vi "OE2052_USB_Query Data.vi"(0 "VISA resource name":refnum<visa-resource-name>, 11 "Error in (no error)":errorcluster caption="error out（no error）") -> (3 "Buffer Count":u8, 4 "VISA resource  out":refnum<visa-resource-name>, 6 "Parameter Values":T1, 8 "Total Data Array":dbl[][](array[numeric]), 10 "Output String":string, 14 "A&B_PLL&Overload":T2, 15 "Error out":errorcluster caption="error out")   [LabVIEW 2011]
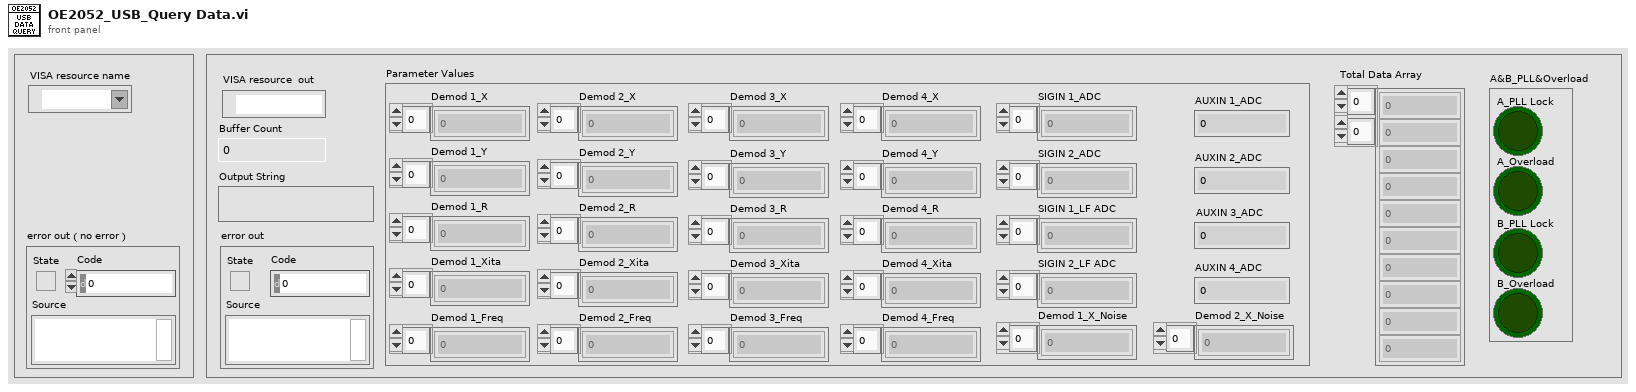
[diagram p1: front panel]
types:
  T1 = cluster{"Demod 1_X":dbl[], "Demod 1_Y":dbl[], "Demod 1_R":dbl[], "Demod 1_Xita":dbl[], "Demod 1_Freq":dbl[], "Demod 2_X":dbl[], "Demod 2_Y":dbl[], "Demod 2_R":dbl[], "Demod 2_Xita":dbl[], "Demod 2_Freq":dbl[], "Demod 3_X":dbl[], "Demod 3_Y":dbl[], "Demod 3_R":dbl[], "Demod 3_Xita":dbl[], "Demod 3_Freq":dbl[], "Demod 4_X":dbl[], "Demod 4_Y":dbl[], "Demod 4_R":dbl[], "Demod 4_Xita":dbl[], "Demod 4_Freq":dbl[], "SIGIN 1_ADC":dbl[], "SIGIN 2_ADC":dbl[], "SIGIN 1_LF ADC":dbl[], "SIGIN 2_LF ADC":dbl[], "AUXIN 1_ADC":dbl, "AUXIN 2_ADC":dbl, "AUXIN 3_ADC":dbl, "AUXIN 4_ADC":dbl, "Demod 1_X_Noise":dbl[], "Demod 2_X_Noise":dbl[]}
  T2 = cluster{"A_PLL Lock":bool, "A_Overload":bool, "B_PLL Lock":bool, "B_Overload":bool}
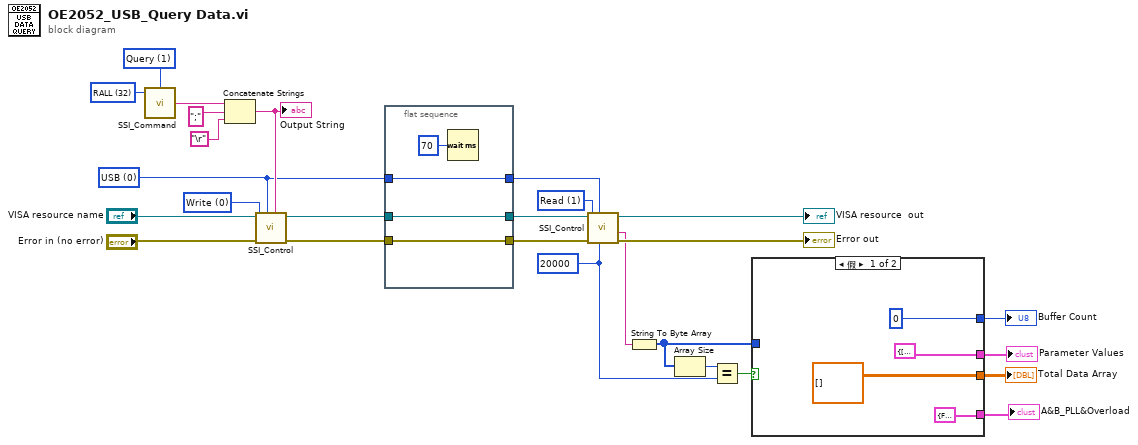
[diagram p0: block diagram]
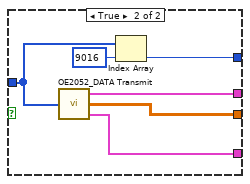
[diagram p2: hidden frame]
diagram:
  w3 = u16 0 items=["USB"=0, "RS232"=1, "Ethernet"=3] ("Remote Mode")
  w14 = u32 20000 ("Number of bytes")
  w17 = u16 1 items=["Write", "Read"] ("Control")
  w19 = u16 0 items=["Write", "Read"] ("Control")
  w24 = u16 32 items=["ISRC", "IGND", "ICPL", "ILIN", "PHAS", "FMOD", "RSLP", "FREQ", "SWPT", "SLLM", "SULM", "SSLL", "SSLG", "STLM", "SWRM", "IRNG", "SENS", "RMOD", "OFLT", "OFSL", "SYNC", "DMOD", "HARM", "DARB", "SWVT", "SLVL", "SVLL", "SVUL", "SVSL", "SVSG", "SVTM", "SVRM", "RALL", "SNAP", "OUTP", "OAUX", "COUT", "CAUX", "COFP", "CEXP", "FPOP", "OEXP", "*IDN", "*RST", "OVLD", "INOV", "GNOV", "*PLL", "SSET", "RSET", "AGAN", "APHS", "ARSV", "ASCL", "EQCD", "EQCS", "SPED", "SRAT", "SLEN", "SSLE", "STRG", "SPRM", "STRD", "PAUS", "RSET", "SPTS", "TRCA", "TEMP", "RSTU", "INHZ", "DEQU", "SADD", "ARNG", "CSPE", "ISRCD", "IGNDD", "ICPLD", "ILIND", "PHASD", "FMODD", "RSLPD", "FREQD", "SWPTD", "SLLMD", "SULMD", "SSLLD", "SSLGD", "STLMD", "SWRMD", "SENSD", "RMODD", "OFLTD", "OFSLD", "SYNCD", "HARMD", "EQCDD", "EQCSD", "SNAPD", "OUTPD", "SWVTD", "SLVLD", "SVLLD", "SVULD", "SVSLD", "SVSGD", "SVTMD", "SVRMD", "SVDCD", "ARSVD", "AGAND", "APHSD", "ASCLD", "FPOPD", "CAUXD", "OEXPD", "SPEDD", "SRATD", "SLEND", "SSLED", "STRGD", "SPRMD", "STRDD", "PAUSD", "RESTD", "SPTSD", "TRCAD", "*IDND", "*RSTD", "INOVD", "GNOVD", "*PLLD", "SSETD", "RSETD", "RALLD"] ("Command Type")
  w22 = u16 1 items=["Set", "Query"] ("Opera")
  n1 = call "SSI_Command.vi"("Opera"=w22, "Command Type"=w24) -> ("Output string"=w25:string)  [unwired: 2 in]
  n2 = Concatenate Strings(w25, ";" ("字符串"), "\r") -> (w27:string)
  "Output String" <- w27
  n3 = call "SSI_Control.vi"("Write Buffer"=w27, "Remote Mode"=w3, "Error in (no error)"="Error in (no error)", "Control"=w19, "VISA resource name"="VISA resource name") -> ("Error out"=w7:errorcluster, "VISA resource  out"=w8:refnum<visa-resource-name>)  [unwired: 3 in, 2 out]
  n4 = flat-sequence {
    tunnel: [w30] -> w9
    tunnel: w3 -> [w30]
    tunnel: [w29] -> w5
    tunnel: w8 -> [w29]
    tunnel: [w28] -> w6
    tunnel: w7 -> [w28]
    frame #0 {
      n5 = Wait (ms)(milliseconds to wait=u32 70 ("等待时间（毫秒）")) -> ()  [unwired: 1 out]
    }
  }
  n6 = call "SSI_Control.vi"("Number of bytes"=w14, "Remote Mode"=w9, "Error in (no error)"=w6, "Control"=w17, "VISA resource name"=w5) -> ("Error out"=→"Error out":errorcluster, "Read Buffer"=w15:string, "VISA resource  out"=→"VISA resource  out":refnum<visa-resource-name>)  [unwired: 3 in, 1 out]
  n7 = String To Byte Array(string=w15) -> (unsigned byte array=w10:u8[])
  n8 = Array Size(array=w10) -> (size(s)=w11:i32)
  n9 = Equal?(x=w11, y=w14) -> (x = y?=w12:bool)
  n10 = case shown="假" w12 {
    tunnel: [u8 0 w40] -> w13
    tunnel: w10 -> [_ w39]
    tunnel: [dbl[][] [] ("Total Data Array") w38] -> w4
    tunnel: [T2 {"A_PLL Lock"=FALSE, "A_Overload"=FALSE, "B_PLL Lock"=FALSE, "B_Overload"=FALSE} ("A&B_PLL&Overload") w37] -> w2
    tunnel: [T1 {"Demod 1_X"=[], "Demod 1_Y"=[], "Demod 1_R"=[], "Demod 1_Xita"=[], "Demod 1_Freq"=[], "Demod 2_X"=[], "Demod 2_Y"=[], "Demod 2_R"=[], "Demod 2_Xita"=[], "Demod 2_Freq"=[], "Demod 3_X"=[], "Demod 3_Y"=[], "Demod 3_R"=[], "Demod 3_Xita"=[], "Demod 3_Freq"=[], "Demod 4_X"=[], "Demod 4_Y"=[], "Demod 4_R"=[], "Demod 4_Xita"=[], "Demod 4_Freq"=[], "SIGIN 1_ADC"=[], "SIGIN 2_ADC"=[], "SIGIN 1_LF ADC"=[], "SIGIN 2_LF ADC"=[], "AUXIN 1_ADC"=0.0, "AUXIN 2_ADC"=0.0, "AUXIN 3_ADC"=0.0, "AUXIN 4_ADC"=0.0, "Demod 1_X_Noise"=[], "Demod 2_X_Noise"=[]} ("Parameter Values") w36] -> w1
    frame False {
    }
    frame True {
      n11 = call "OE2052_DATA Transmit.vi"("Input Data"=w39) -> ("Parameter Values"=w36:T1, "Total Data Array"=w38:dbl[][], "A&B_PLL&Overload"=w37:T2)
      n12 = Index Array(array=w39, index=9016 ("索引")) -> (element=w40:u8)
    }
  }
  "Buffer Count" <- w13
  "Total Data Array" <- w4
  "A&B_PLL&Overload" <- w2
  "Parameter Values" <- w1
